vi "Serialize.vi"(8 "error in":errorcluster, 11 "Data":T1) -> (0 "error out":errorcluster, 3 "XMLString":string)   [LabVIEW 2021, in "ProligentXMLGenerator.lvlib" / "Datawarehouse.lvclass"]
uses:
  Datawarehouse.lvclass
  Datawarehouse.lvclass/Datawarehouse.ctl
  Failure/Defect/Defect.lvclass
  <vilib>/xml/NI_XML.lvlib
  ProcessRun/ProcessRun.lvclass
  Base/DOMSupport/DOMSupport.lvlib
  <resource>/objmgr/DOMUserDefRef.rc
  <vilib>/xml/Close Reference(Node).vi
  ProductUnit/ProductUnit.lvclass
  Base/DateTime/DateTime.lvclass
  C:/Projects/proligent-xml-generator-labview/src/ProligentXMLGenerator/Base/Attribute/Attribute.lvclass
  C:/Projects/proligent-xml-generator-labview/src/ProligentXMLGenerator/Base/DateTime/DateTime.lvclass
  Base/NonEmptyString_2000/NonEmptyString_2000.lvclass
  C:/Projects/proligent-xml-generator-labview/src/ProligentXMLGenerator/Base/NonEmptyString/NonEmptyString.lvclass
  C:/Projects/proligent-xml-generator-labview/src/ProligentXMLGenerator/Base/String/String.lvclass
  C:/Projects/proligent-xml-generator-labview/src/ProligentXMLGenerator/Base/NonEmptyString_2000/NonEmptyString_2000.lvclass
  Base/NonEmptyString_448/NonEmptyString_448.lvclass
  C:/Projects/proligent-xml-generator-labview/src/ProligentXMLGenerator/Base/NonEmptyString_448/NonEmptyString_448.lvclass
  Data.ctl
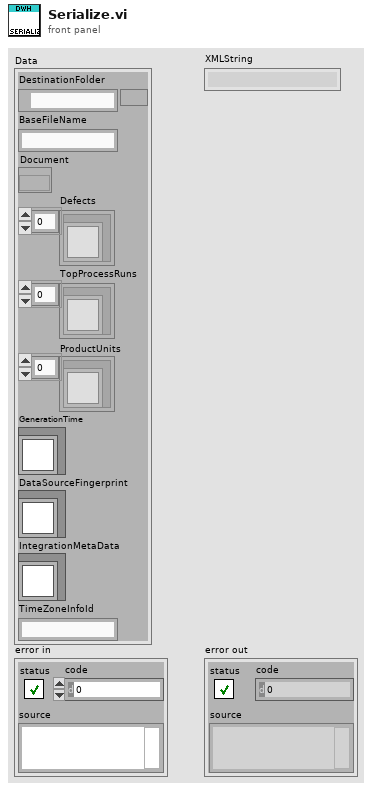
[diagram p1: front panel]
types:
  T1 = typedef "ProligentXMLGenerator.lvlib/Datawarehouse.lvclass/Data.ctl" = cluster{"DestinationFolder":path, "BaseFileName":string, "Document":refnum<k20>, "Defects":refnum<class "Defect.lvclass">[], "TopProcessRuns":refnum<class "ProcessRun.lvclass">[], "ProductUnits":refnum<class "ProductUnit.lvclass">[], "GenerationTime":refnum<class "DateTime.lvclass">, "DataSourceFingerprint":refnum<class "NonEmptyString_448.lvclass">, "IntegrationMetaData":refnum<class "NonEmptyString_2000.lvclass">, "TimeZoneInfoId":string}
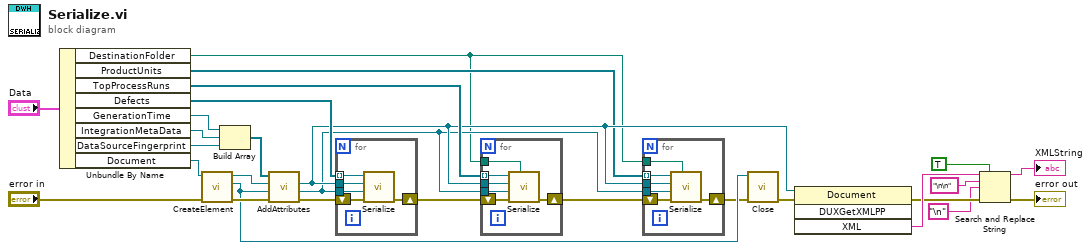
[diagram p0: block diagram]
diagram:
  n1 = Unbundle By Name("Data") -> ("DestinationFolder"=w1:path, "ProductUnits"=w2:refnum<class "ProductUnit.lvclass">[], "TopProcessRuns"=w24:refnum<class "ProcessRun.lvclass">[], "Defects"=w26:refnum<class "Defect.lvclass">[], "GenerationTime"=w20:refnum<class "DateTime.lvclass">, "IntegrationMetaData"=w19:refnum<class "NonEmptyString_2000.lvclass">, "DataSourceFingerprint"=w18:refnum<class "NonEmptyString_448.lvclass">, "Document"=w25:refnum<k20>)
  n2 = call "CreateElement.vi"("error in"="error in", "Document in"=w25) -> ("error out"=w22:errorcluster, "Element"=w16:refnum<k20>, "Document out"=w15:refnum<k20>)  [unwired: 7 in]
  n3 = Build Array(w20, w19, w18) -> (w17:refnum<class "Attribute.lvclass">[])
  n4 = call "AddAttributes.vi"("error in"=w22, "OwningElement in"=w16, "Document in"=w15, "Attributes"=w17) -> ("error out"=w21:errorcluster, "OwningElement out"=w4:refnum<k20>, "Document out"=w5:refnum<k20>)  [unwired: 5 in]
  n5 = for {
    tunnel: w26 -> [w33] mode=indexing
    tunnel: w4 -> [w31]
    tunnel: w5 -> [w32]
    shift-right: [w29] -> w23
    shift-left: w21 -> [w30]
    n6 = call "Serialize.vi"("error in"=w30, "OwningElement in"=w31, "Document in"=w32, "Defect in"=w33) -> ("error out"=w29:errorcluster)  [unwired: 4 in, 3 out]
  }
  n7 = for {
    tunnel: w24 -> [w39] mode=indexing
    tunnel: w4 -> [w37]
    tunnel: w5 -> [w38]
    shift-right: [w35] -> w6
    shift-left: w23 -> [w36]
    tunnel: w1 -> [w34]
    n8 = call "Serialize.vi"("DestinationFolder"=w34, "error in"=w36, "OwningElement in"=w37, "Document in"=w38, "ProcessRun in"=w39) -> ("error out"=w35:errorcluster)  [unwired: 3 in, 3 out]
  }
  n9 = for {
    tunnel: w2 -> [w45] mode=indexing
    tunnel: w4 -> [w43]
    tunnel: w5 -> [w44]
    shift-right: [w41] -> w3
    shift-left: w6 -> [w42]
    tunnel: w1 -> [w40]
    n10 = call "Serialize.vi"("DestinationFolder"=w40, "error in"=w42, "OwningElement in"=w43, "Document in"=w44, "ProductUnit in"=w45) -> ("error out"=w41:errorcluster)  [unwired: 3 in, 3 out]
  }
  n11 = call-poly <vilib>:"Close.vi"("error in (no error)"=w3, "node"=w16) -> ("error out"=w9:errorcluster)  [unwired: 7 in]
  n12 = invoke on="Invoke Node" class="Document" method="DUXGetXMLPP"(reference=w5, error in=w9) -> (error out=w13:errorcluster, "XML"=w14:string)  [unwired: 2 in, 2 out]
  n13 = Search and Replace String(replace all?=TRUE ("replace all? (F)"), input string=w14, search string="\n\n", replace string="\n", error in=w13) -> (result string=→"XMLString":string, error out=→"error out":errorcluster)  [unwired: 3 in, 2 out]
